vi "Self-Alignment Operations.vi"(8 "error in (no error)":errorcluster, 10 "Operation (Start)":i32(ring) items=["Start", "Stop", "Abort"], 11 "VISA resource name":refnum<visa-resource-name>) -> (0 "error out":errorcluster, 3 "VISA resource name out":refnum<visa-resource-name>)   [LabVIEW 2020, in "Rohde&Schwarz CMXP Base.lvlib"]
doc: "Starts the measurement procedure.\n\nAttributes:\nRSCMXPBASE_ATTR_MEASURMENT_START\nRSCMXPBASE_ATTR_MEASURMENT_STOP\nRSCMXPBASE_ATTR_MEASURMENT_ABORT\n\nRemote-control commands:\nINITiate:BASE:SALignment\nSTOP:BASE:SALignment\nABORt:BASE:SALignment"
uses:
  <instrlib>/Rohde&Schwarz CMXP Base/Rohde&Schwarz CMXP Base.lvlib
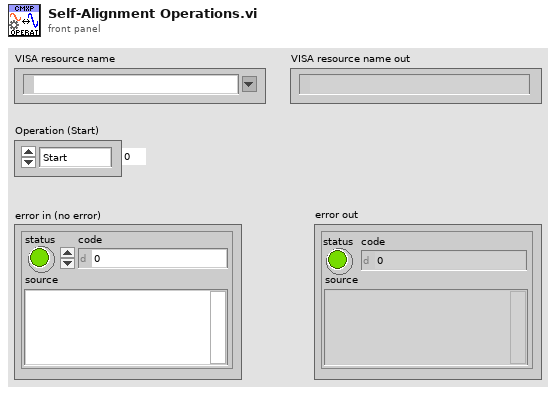
[diagram p1: front panel]
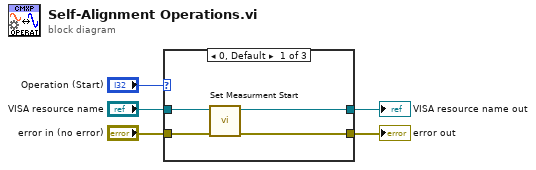
[diagram p0: block diagram]
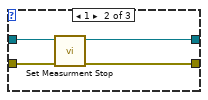
[diagram p2: hidden frame]
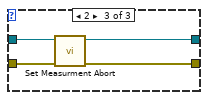
[diagram p3: hidden frame]
diagram:
  n1 = case shown="0, Default" "Operation (Start)" {
    tunnel: "error in (no error)" -> [w9 w13 w17]
    tunnel: "VISA resource name" -> [w8 w12 w16]
    tunnel: [w7 w11 w15] -> w3
    tunnel: [w6 w10 w14] -> w2
    frame 0, Default {
      n2 = call "Set Measurment Start"("error in (no error)"=w9, "instrument handle"=w8) -> ("error out"=w7:errorcluster, "instrument handle out"=w6:refnum<visa-resource-name>)  [unwired: 8 in]
    }
    frame 1 {
      n3 = call "Set Measurment Stop"("error in (no error)"=w13, "instrument handle"=w12) -> ("error out"=w11:errorcluster, "instrument handle out"=w10:refnum<visa-resource-name>)  [unwired: 8 in]
    }
    frame 2 {
      n4 = call "Set Measurment Abort"("error in (no error)"=w17, "instrument handle"=w16) -> ("error out"=w15:errorcluster, "instrument handle out"=w14:refnum<visa-resource-name>)  [unwired: 8 in]
    }
  }
  "error out" <- w3
  "VISA resource name out" <- w2
